vi "Get single frame from buffer.vi"(8 "error in (no error)":errorcluster, 11 "uCAN in":refnum<class "uCAN.lvclass">) -> (0 "error out":errorcluster, 2 "Frame":T1 {"Data" format="%.0x"}, 3 "uCAN out":refnum<class "uCAN.lvclass">)   [LabVIEW 2021, in "uCanDriver.lvlib" / "uCAN.lvclass"]
uses:
  uCAN.lvclass
  typedefs/frame.ctl
  uCAN.lvclass/uCAN.ctl
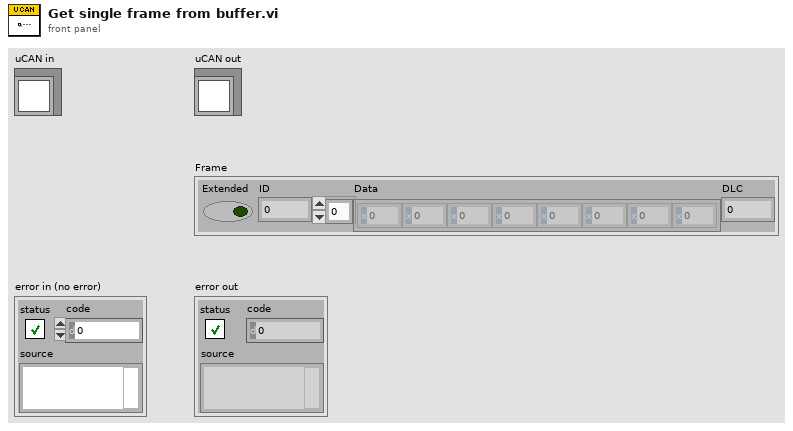
[diagram p1: front panel]
types:
  T1 = typedef "uCanDriver.lvlib/uCAN.lvclass/frame.ctl" = cluster{"Extended":bool, "ID":u32, "Data":u8[], "DLC":u8}
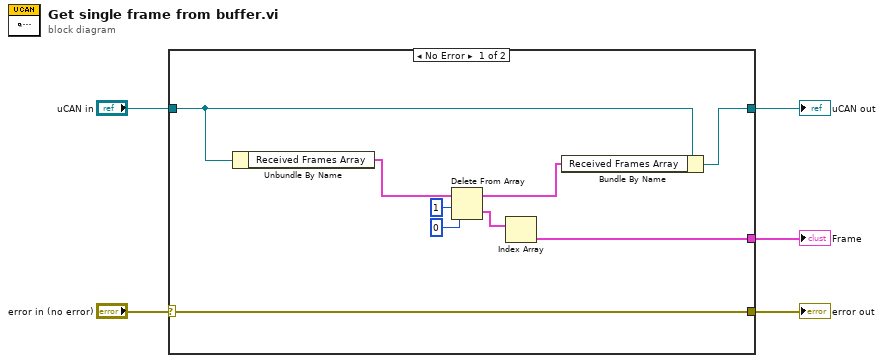
[diagram p0: block diagram]
diagram:
  n1 = case shown="No Error" "error in (no error)" {
    selector: "error in (no error)" -> [w14 w16]
    tunnel: [w14 w16] -> w4
    tunnel: [w12 w15] -> w2
    tunnel: "uCAN in" -> [w13 w15]
    tunnel: [w6 _] -> w1
    frame No Error {
      n2 = Unbundle By Name(w13) -> ("Received Frames Array"=w11:T1[])
      n3 = Delete From Array(array=w11, length=1, index=0) -> (deleted portion=w7:T1[], array with subset deleted=w10:T1[])
      n4 = Index Array(array=w7) -> (element=w6:T1)  [unwired: 1 in]
      n5 = Bundle By Name(cluster=w13, "Received Frames Array"=w10) -> (w12:refnum<class "uCAN.lvclass">)
    }
    frame Error {
    }
  }
  "error out" <- w4
  "uCAN out" <- w2
  "Frame" <- w1
